vi "Init.vi"(8 "error in (no error)":errorcluster, 9 "N5222A Cfg":T1={"ResourceName"="", "Enable"=FALSE, "Channel"=1, "CalFileName"="", "MeasName"="", "TempDatFile"="", "Power, dBm"=-30.0, "NumPoints"=201, "Start Freq, Hz"=5000000000.0, "Stop Freq, Hz"=6000000000.0, "NumAverages"=20, "Sweep Type"=0, "IF Bandwidth"=0.0} {"Sweep Type" items=["Linear Frequency", "Log Frequency", "Power Sweep", "CW Time"]; "Stop Freq, Hz" format="%_3p"; "Start Freq, Hz" format="%_3p"}, 11 "N5222A PNA in":refnum<class "N5222A PNA.lvclass">) -> (0 "error out":errorcluster, 3 "N5222A PNA out":refnum<class "N5222A PNA.lvclass">)   [LabVIEW 2019, in "N5222A PNA.lvclass"]
uses:
  N5222A PNA.lvclass
  N5222AConfig.ctl
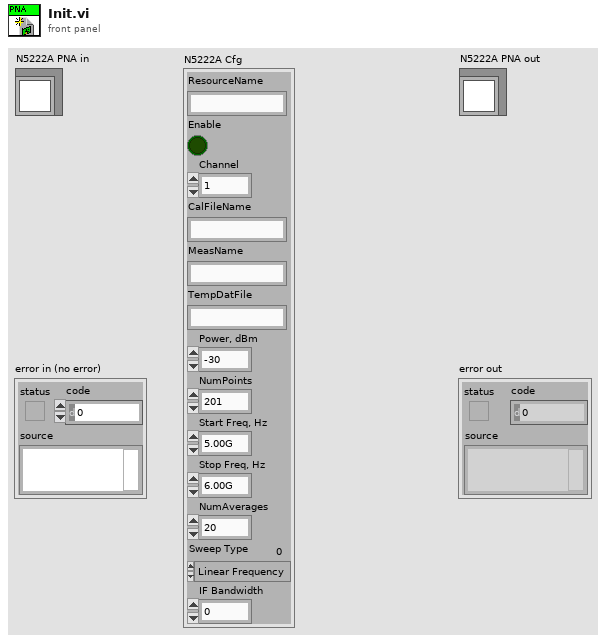
[diagram p1: front panel]
types:
  T1 = typedef "N5222AConfig.ctl" = cluster{"ResourceName":string, "Enable":bool, "Channel":i32, "CalFileName":string, "MeasName":string, "TempDatFile":string, "Power, dBm":dbl, "NumPoints":i32, "Start Freq, Hz":dbl, "Stop Freq, Hz":dbl, "NumAverages":i32, "Sweep Type":i32, "IF Bandwidth":dbl}
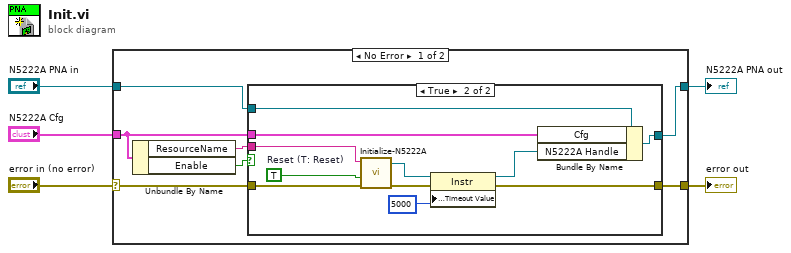
[diagram p0: block diagram]
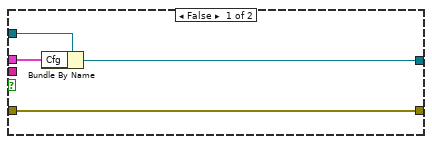
[diagram p2: hidden frame]
diagram:
  n1 = case shown="No Error" "error in (no error)" {
    selector: "error in (no error)" -> [w7 w29]
    tunnel: [w6 w29] -> w4
    tunnel: [w10 w28] -> w2
    tunnel: "N5222A PNA in" -> [w11 w28]
    tunnel: "N5222A Cfg" -> [w9 _]
    frame No Error {
      n2 = Unbundle By Name(w9) -> ("ResourceName"=w12:string, "Enable"=w8:bool)
      n3 = case shown="True" w8 {
        tunnel: w12 -> [_ w27]
        tunnel: w7 -> [w16 w26]
        tunnel: w11 -> [w14 w25]
        tunnel: [w13 w24] -> w10
        tunnel: w9 -> [w15 w23]
        tunnel: [w16 w19] -> w6
        frame False {
          n4 = Bundle By Name(cluster=w14, "Cfg"=w15) -> (w13:refnum<class "N5222A PNA.lvclass">)
        }
        frame True {
          w22 = TRUE  # Reset (T: Reset)
          n5 = call <instrlib>:"Initialize-N5222A.vi"("error in (no error)"=w26, "Reset (T: Reset)"=w22, "Instrument Resource Name"=w27) -> ("error out"=w20:errorcluster, "dup VISA session"=w17:refnum<visa-resource-name>)  [unwired: 7 in]
          n6 = property class="Instr"(reference=w17, error in=w20, "General Settings:Timeout Value"=u32 5000 ("Tmo Value")) -> (reference out=w18:refnum<visa-resource-name>, error out=w19:errorcluster)
          n7 = Bundle By Name(cluster=w25, "Cfg"=w23, "N5222A Handle"=w18) -> (w24:refnum<class "N5222A PNA.lvclass">)
        }
      }
    }
    frame Error {
    }
  }
  "error out" <- w4
  "N5222A PNA out" <- w2
